vi "Output.vi"(10 "Msg Output":refnum<class "Msg Output.lvclass">) -> ()   [LabVIEW 2025, in "jettl.lvlib" / "Stopped Msg.lvlib" / "Stopped Msg Output.lvclass"]
uses:
  Stopped Msg Output.lvclass
  Stopped Msg Output.lvclass/Stopped Msg Output.ctl
  Msg Output/Msg Output.lvclass
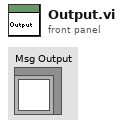
[diagram p1: front panel]
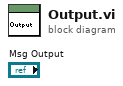
[diagram p0: block diagram]
diagram:
